vi "RemoveGObject.vi"(0 "__args":cluster{"targetVi":string, "uid":i32}) -> (1 "__return":i32, 2 "__errStatus":bool, 3 "__errCode":i32, 4 "__errSource":string)   [LabVIEW 2013]
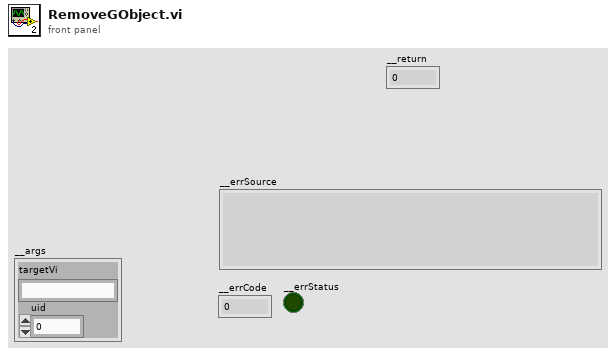
[diagram p1: front panel]
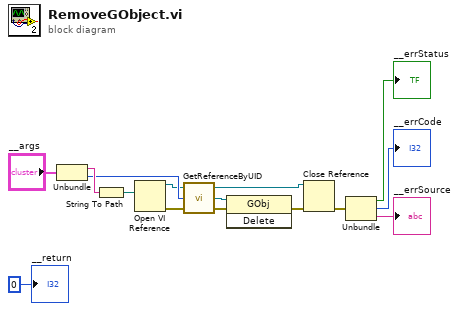
[diagram p0: block diagram]
diagram:
  n1 = Unbundle("__args") -> ("targetVi"=w11:string, "uid"=w8:i32)
  n2 = String To Path(string=w11) -> (path=w10:path)
  n3 = Open VI Reference(vi path=w10) -> (vi reference=w7:refnum<vi>, error out=w6:errorcluster)  [unwired: 5 in]
  n4 = call "GetReferenceByUID.vi"("error in (no error)"=w6, "UID"=w8, "targetVI"=w7) -> ("error out"=w3:errorcluster, "refNum"=w5:refnum<vi>, "dup targetVI"=w4:refnum<vi>)
  n5 = invoke class="GObj" method="Delete"(reference=w5, error in=w3) -> (error out=w1:errorcluster)  [unwired: 1 in, 2 out]
  n6 = Close Reference(reference=w4, error in (no error)=w1) -> (error out=w2:errorcluster)
  n7 = Unbundle(w2) -> ("status"=→"__errStatus":bool, "code"=→"__errCode":i32, "source"=→"__errSource":string)
  "__return" <- 0
